vi "加标回收启动 (子VI).vi"(10 "加标体积":dbl format="%#_13g", 11 "启动参数":T1(ring)=enum."CODCr") -> (0 "error out":T2={"status"=FALSE, "代码"=4, "source"=""} caption="错误输出" {"代码" items=["执行成功"=1, "执行失败，但不知道原因"=2, "命令请求条件错误"=3, "通讯超时"=4, "系统繁忙不能执行"=5, "系统故障"=6, "没有数据"=100]})   [LabVIEW 2016, in "MB SLAVE.lvlib"]
uses:
  MB SLAVE.lvlib
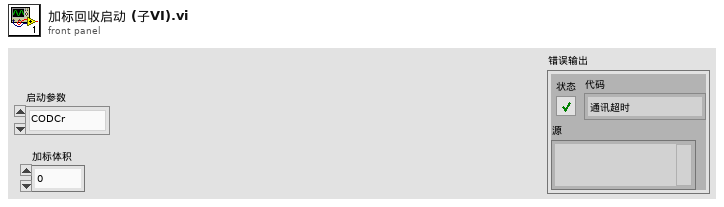
[diagram p1: front panel]
types:
  T1 = enum16{"未选择", "CODMn", "氨氮", "总磷", "总氮", "CODCr"}
  T2 = cluster{"status":bool, "代码":u16, "source":string}
  T3 = typedef "测试子流程.ctl" = enum16{"加标回收（启动采配水）", "加标回收（不启动采配水）", "水样测试（启动采配水）", "水样测试（不启动采配水）", "平行样测试（启动采配水）", "平行样测试（不启动采配水）", "集成干预测试"}
  T4 = typedef "质控slave id.ctl" = enum16{"null", "氨氮", "总磷", "总氮", "CODMn", "CODCr", "氟化物"}
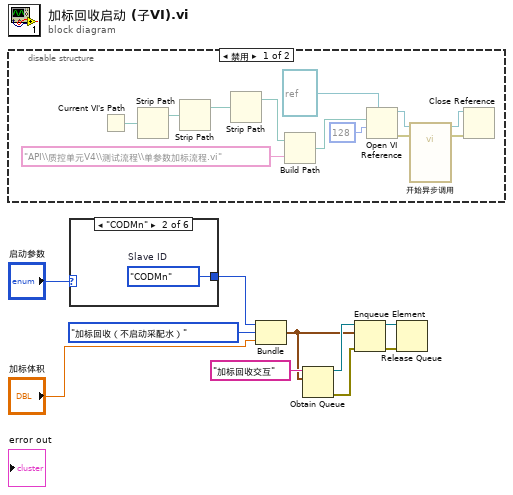
[diagram p0: block diagram]
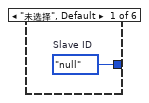
[diagram p3: hidden frame]
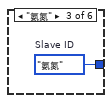
[diagram p4: hidden frame]
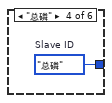
[diagram p5: hidden frame]
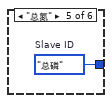
[diagram p6: hidden frame]
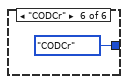
[diagram p7: hidden frame]
diagram:
  n1 = disable-structure shown="禁用" {
    frame Disabled {
      n2 = Current VI's Path() -> (path=w22:path)
      n3 = Strip Path(path=w22) -> (stripped path=w13:path)  [unwired: 1 out]
      n4 = Strip Path(path=w13) -> (stripped path=w12:path)  [unwired: 1 out]
      n5 = Strip Path(path=w12) -> (stripped path=w20:path)  [unwired: 1 out]
      n6 = Build Path(base path=w20, name or relative path="API\\质控单元V4\\测试流程\\单参数加标流程.vi" ("名称或相对路径")) -> (appended path=w14:path)
      n7 = Open VI Reference(type specifier VI Refnum (for type only)=refnum<vi> refnum, vi path=w14, options=128 ("选项")) -> (vi reference=w16:refnum<vi>, error out=w17:errorcluster)  [unwired: 3 in]
      n8 = call-by-ref "开始异步调用"(reference=w16, error in=w17) -> (reference out=w18:refnum<vi>, error out=w19:errorcluster)  [unwired: 12 in]
      n9 = Close Reference(reference=w18, error in (no error)=w19) -> ()  [unwired: 1 out]
    }
    frame Enabled {
    }
  }
  n10 = case shown="\"CODMn\"" "启动参数" {
    tunnel: [w23 w24 w25 w26 w27 质控slave_id."CODCr" ("Slave ID")] -> w4
    frame "未选择", Default {
      w23 = 质控slave_id."null"  # Slave ID
    }
    frame "CODMn" {
      w24 = 质控slave_id."CODMn"  # Slave ID
    }
    frame "氨氮" {
      w25 = 质控slave_id."氨氮"  # Slave ID
    }
    frame "总磷" {
      w26 = 质控slave_id."总磷"  # Slave ID
    }
    frame "总氮" {
      w27 = 质控slave_id."总磷"  # Slave ID
    }
    frame "CODCr" {
    }
  }
  n11 = Bundle("Slave ID"=w4, "流程参数"=测试子流程."加标回收（不启动采配水）", "加标体积"="加标体积") -> (w3:cluster{"Slave ID":T4, "流程参数":T3, "加标体积":dbl})  [unwired: 1 in]
  n12 = Obtain Queue(name (unnamed)="加标回收交互" ("名称（未命名）"), element data type=w3) -> (queue out=w8:refnum<queue>, error out=w7:errorcluster)  [unwired: 3 in, 1 out]
  n13 = Enqueue Element(queue=w8, element=w3, error in (no error)=w7) -> (queue out=w6:refnum<queue>, error out=w5:errorcluster)  [unwired: 1 in, 1 out]
  n14 = Release Queue(queue=w6, error in (no error)=w5) -> ()  [unwired: 1 in, 3 out]
